vi "Kinect Demo.vi"(8 "stop":bool) -> (1 "average Z":dbl, 2 "average X":dbl, 3 "average Y":dbl)   [LabVIEW 2011, in "Kinect_API.lvlib"]
uses:
  Kinect_API.lvlib
  <vilib>/Platform/TimedLoop/XDataNode/timing_clust.ctl
  <vilib>/Platform/TimedLoop/XDataNode/nitl_modes.ctl
  <vilib>/Platform/TimedLoop/XDataNode/wakeup.ctl
  average Y.vi
  <vilib>/Platform/TimedLoop/XDataNode/XDataNode.xnode
  <vilib>/Platform/TimedLoop/XDataNode/XDNodeRunTimeDep.lvlib
panel:
  in  "Wall-Threshold":i32=150
  in  "stop 2":bool
  out "click 2":bool
  out "Area":i32
  in  "Y-Threshold":i32=150
  out "Depth 2":T1(plugin-control)
  in  "Replace with?":i32=60000
  in  "Far object filter":i32(slide)=26869 scale=0.0..4305.0
  out "Depth Image Pixels (U16)":i32[][](array[numeric])
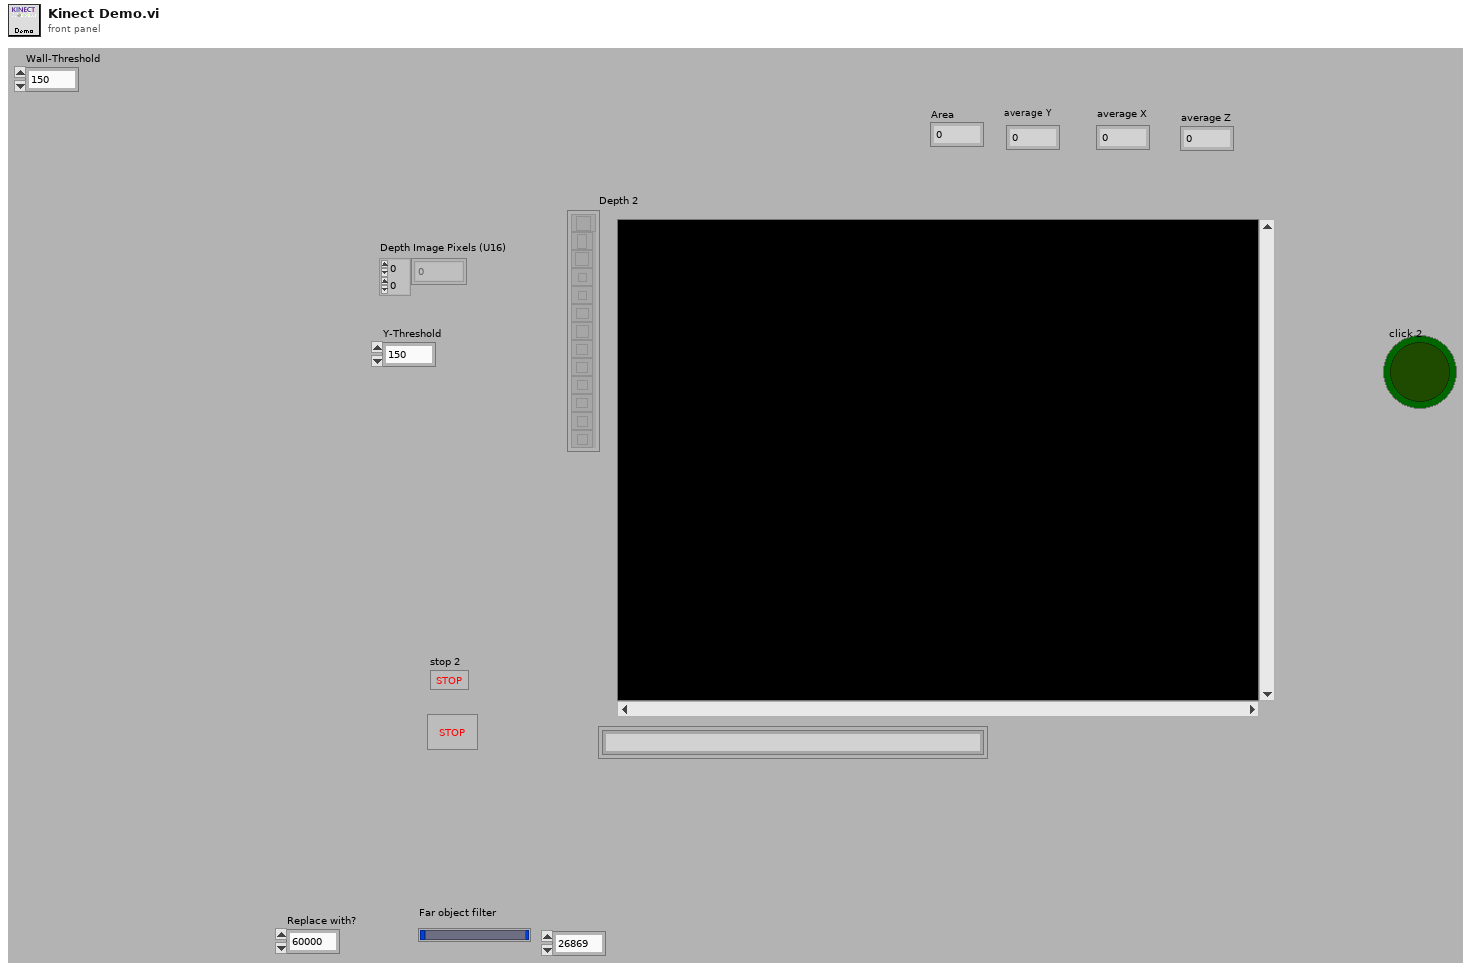
[diagram p1: front panel]
types:
  T1 = typedef "IMAQ Image.ctl" = refnum<image>
  T2 = typedef "XDNodeRunTimeDep.lvlib/timing_clust.ctl" = cluster{"Expected End [f-1]":u64, "Actual End [f-1]":u64, "Finished Late? [f-1]":bool, "Expected End [i-1]":u64, "Actual End [i-1]":u64, "Finished Late? [i-1]":bool, "Expected Start [i]":u64, "Actual Start [i]":u64, "Expected Start [f]":u64, "Actual Start [f]":u64, "Source Name":string, "Structure Name":string, "Period":i64, "Deadline":i64, "Offset":i64, "Start":i64, "Priority":i32, "Timeout":i32, "Mode":T3, "Wakeup Reason":T4, "Error":errorcluster, "Source Type":string, "Secondary Source Type":string, "Global End Time":u64, "Global Start Time":u64, "Frame Duration":u64, "Iteration Duration":u64, "Assigned CPU":i32, "I/O Scan Engine Mode":u32}
  T3 = typedef "XDNodeRunTimeDep.lvlib/nitl_modes.ctl" = enum32{"No Change", "Process missed periods, maintain original phase", "Discard missed periods, maintain original phase", "Process missed periods, ignore original phase", "Discard missed periods, ignore original phase"}
  T4 = typedef "XDNodeRunTimeDep.lvlib/wakeup.ctl" = enum32{"Normal", "Aborted", "Asynchronous wakeup", "Timing source error", "Timed loop error", "Timeout"}
  T5 = cluster{"queue out":refnum<queue>, "queue out":refnum<queue>}
  T6 = cluster{"new reference":refnum<k24>, "DepthStream":refnum<k24>, "VideoStream":refnum<k24>, "Event Callback":refnum<k27>, "Event Callback":refnum<k27>}
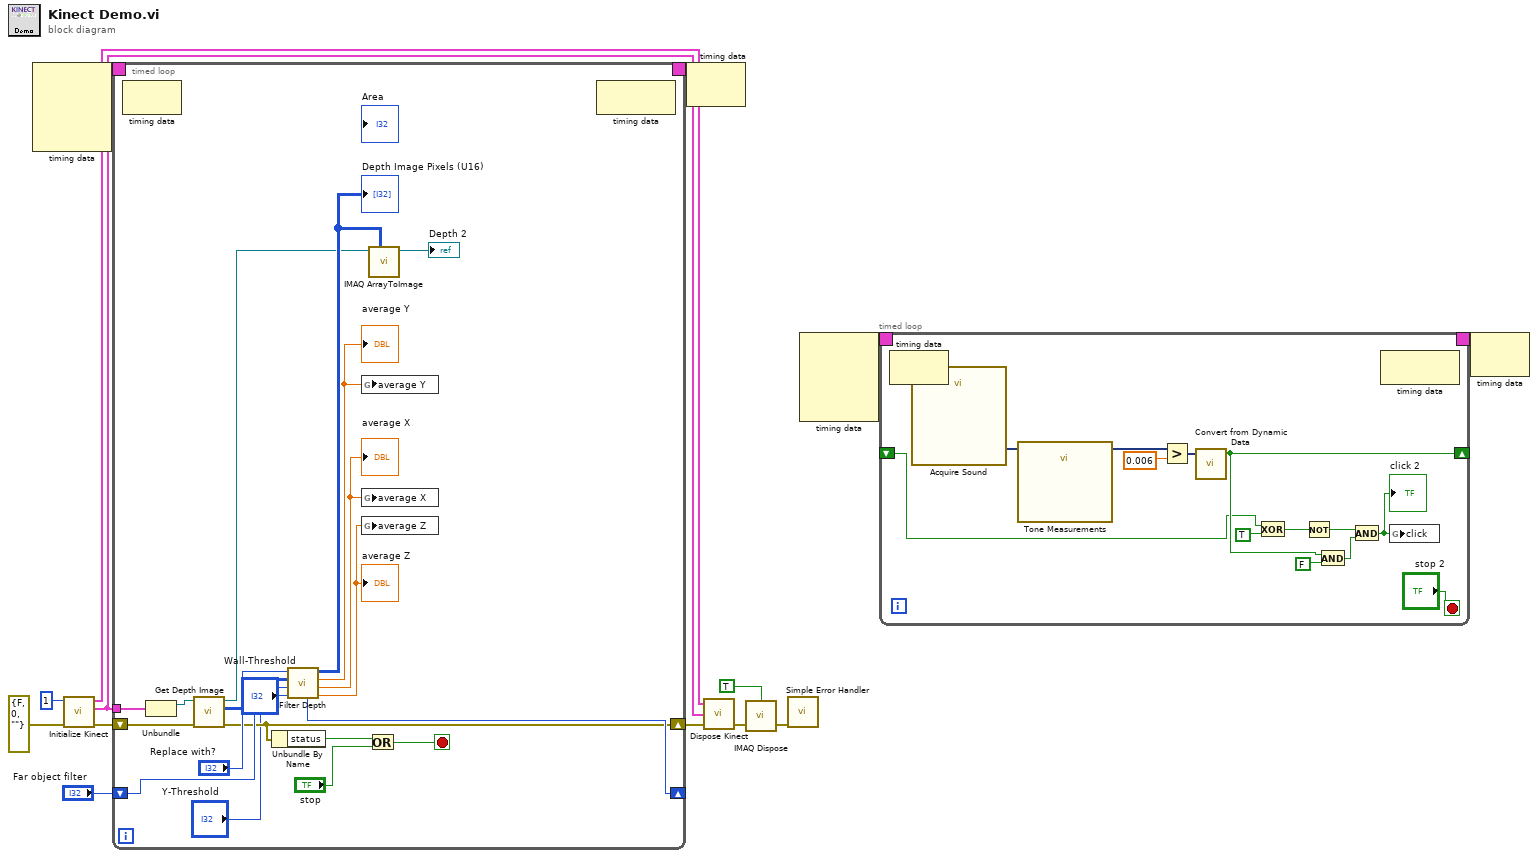
[diagram p0: block diagram]
diagram:
  n1 = node-c288() -> (w4:T2)  [unwired: 4 in]
  n2 = call "Initialize Kinect.vi"("error in (no error)"=errorcluster {"status"=FALSE, "code"=0, "source"=""}, "Buffer Size"=1) -> ("error out"=w12:errorcluster, "Queues Out"=w8:T5, "References"=w13:T6)  [unwired: 7 in]
  n3 = timed-loop {
    tunnel: w8 -> [w33]
    shift-right: [w21] -> w11
    shift-left: w12 -> [w29]
    shift-right: [w22] -> _
    shift-left: "Far object filter" -> [w23]
    timing: w4 -> [_]
    timing-out: [_] -> w3
    stop <- w30 stop-if-true
    n4 = node-c288() -> ()  [unwired: 1 in, 1 out]
    n5 = Unbundle(w33) -> ("queue out"=w28:refnum<queue>)  [unwired: 1 out]
    n6 = call "Get Depth Image.vi"("error in (no error)"=w29, "queue in"=w28) -> ("error out"=w21:errorcluster, "Depth Image Pixels (U16)"=w25:u16[][], "Depth Image"=w24:T1)  [unwired: 6 in, 1 out]
    n7 = Unbundle By Name(w21) -> ("status"=w32:bool)
    n8 = call "Filter Depth.vi"("Wall-Threshold"="Wall-Threshold", "Y-Threshold"="Y-Threshold", "Far object filter"=w23, "Depth Image Pixels (U16)"=w25, "Replace with?"="Replace with?") -> ("average Z"=w17:dbl, "average Y"=w18:dbl, "average X"=w19:dbl, "Array"=w27:i32[][], "New far object filter"=w22:i32)  [unwired: 1 in, 1 out]
    "Depth Image Pixels (U16)" <- w27
    "average Y" <- w19
    "average X" <- w18
    "average Z" <- w17
    n9 = global write "average Y.vi" "average Y"(w19) -> ()
    n10 = global write "average Y.vi" "average X"(w18) -> ()
    n11 = global write "average Y.vi" "average Z"(w17) -> ()
    n12 = Or(x=w32, y="stop") -> (x .or. y?=w30:bool)
    n13 = call "IMAQ ArrayToImage"("Image Pixels (U16)"=w27, "Image"=w24) -> ("Image Out"=→"Depth 2":T1)  [unwired: 8 in, 1 out]
    n14 = node-c288() -> ()  [unwired: 1 in, 1 out]
  }
  n15 = node-c288(w3) -> ()  [unwired: 1 out]
  n16 = call "Dispose Kinect.vi"("error in (no error)"=w11, "Queues In"=w8, "References"=w13) -> ("error out"=w6:errorcluster)  [unwired: 2 in]
  n17 = call "IMAQ Dispose"("All Images? (No)"=TRUE, "error in (no error)"=w6) -> ("error out"=w9:errorcluster)  [unwired: 4 in]
  n18 = call <vilib>:"Simple Error Handler.vi"("error in (no error)"=w9) -> ()  [unwired: 4 in, 5 out]
  n19 = node-c288() -> (w2:T2)  [unwired: 4 in]
  n20 = timed-loop {
    shift-right: [w37] -> _
    shift-left: _ -> [w36]
    timing: w2 -> [_]
    timing-out: [_] -> w1
    stop <- "stop 2" stop-if-true
    n21 = node-c288() -> ()  [unwired: 1 in, 1 out]
    n22 = call "Acquire Sound"() -> ("Data"=w47:dynamicdata)  [unwired: 18 in, 1 out]
    n23 = call "Tone Measurements"("Signals"=w47) -> ("Amplitude"=w46:dynamicdata)  [unwired: 9 in, 1 out]
    n24 = Greater?(x=w46, y=0.006) -> (0:w44:dynamicdata)
    n25 = call "Convert from Dynamic Data"("Dynamic Data Type"=w44) -> ("Scalar"=w37:bool)  [unwired: 3 in]
    n26 = Exclusive Or(1:TRUE, 2:w36) -> (0:w41:bool)
    n27 = Not(x=w41) -> (.not. x?=w40:bool)
    n28 = And(x=w37, y=FALSE) -> (x .and. y?=w39:bool)
    n29 = And(x=w40, y=w39) -> (x .and. y?=w38:bool)
    "click 2" <- w38
    n30 = node-c288() -> ()  [unwired: 1 in, 1 out]
    n31 = global write "average Y.vi" "click"(w38) -> ()
  }
  n32 = node-c288(w1) -> ()  [unwired: 1 out]
